vi "Write_LS_Data_without_LS370.vi"(1 "In":T1={"Time"=[], "LI1CH1"=[], "LI1CH2"=[], "LI2CH1"=[], "LI2CH2"=[], "LI3CH1"=[], "LI3CH2"=[], "Field"=[], "N_Level"=[], "H_Level"=[], "Heat_370"=[], "Sorb_Heat"=[], "Still_Heat"=[], "Capacity"=[], "Loss"=[], "Magnet_Temperature"=[], "Lam_Pressure"=[], "Lam_NValve"=[], "370-T1"=[], "370-T2"=[], "370-T3"=[], "370-T4"=[], "370-T5"=[], "370-R1"=[], "370-R2"=[], "370-R3"=[], "370-R4"=[], "370-R5"=[], "372-T1"=[], "372-T2"=[], "372-T3"=[], "372-T4"=[], "372-T5"=[], "372-T6"=[], "372-R1"=[], "372-R2"=[], "372-R3"=[], "372-R4"=[], "372-R5"=[], "372-R6"=[], "Nada"=[nan], "K2440_Res"=[], "K2440_Current"=[], "VTI_Heater"=[], "VTI_NValve"=[], "LS340_Heater"=[], "K6221_Amplitude"=[], "K6221_Frequency"=[], "Cond_Pressure"=[], "Still_Pressure"=[], "FP_Out_Pressure"=[], "Dump_Pressure"=[], "V1"=[], "V2"=[], "V4"=[], "V5"=[], "V9"=[], "Forepump"=[], "Compressor"=[], "K6221_Offset"=[], "BoxTemp"=[], "By"=[], "Bz"=[], "Phi"=[], "heater-recond (%)"=[], "Dewar Pressure "=[], "JT-SP-Control"=[], "350 T1"=[], "350 T2"=[], "350 T3"=[], "350 T4"=[], "350 R1"=[], "350 R2"=[], "350 R3"=[], "350 R4"=[], "Angle"=[], "VTI CH1"=[], "VTI CH2"=[], "VTI CH3"=[], "ColdTrap"=[], "Mischer Pot"=[], "G1 (mbar)"=[], "G3 (mbar) "=[], "G4 (mbar)"=[], "IVC (mbar)"=[], "P2 (mbar) "=[], "Pot mischer (mbar)"=[], "AVS Control Channel (K)"=[], "AVS Control Channel (RES)"=[], "AVS  Channel 5 (RES) "=[], "LI3CH3"=[], "LI3CH4"=[], "LI1CH3"=[], "LI1CH4"=[], "LI2CH3"=[], "LI2CH4"=[], "Volt"=[], "Watt"=[], "Torque Angle"=[], "Dewar heater (W)"=[], "PSU Voltage"=[], "Turbopump"=[], "372-R7"=[], "372-T7"=[], "SIM921 Ch1"=[]}) -> (0 "Out":T1={"Time"=[], "LI1CH1"=[], "LI1CH2"=[], "LI2CH1"=[], "LI2CH2"=[], "LI3CH1"=[], "LI3CH2"=[], "Field"=[], "N_Level"=[], "H_Level"=[], "Heat_370"=[], "Sorb_Heat"=[], "Still_Heat"=[], "Capacity"=[], "Loss"=[], "Magnet_Temperature"=[], "Lam_Pressure"=[], "Lam_NValve"=[], "370-T1"=[], "370-T2"=[], "370-T3"=[], "370-T4"=[], "370-T5"=[], "370-R1"=[], "370-R2"=[], "370-R3"=[], "370-R4"=[], "370-R5"=[], "372-T1"=[], "372-T2"=[], "372-T3"=[], "372-T4"=[], "372-T5"=[], "372-T6"=[], "372-R1"=[], "372-R2"=[], "372-R3"=[], "372-R4"=[], "372-R5"=[], "372-R6"=[], "Nada"=[nan], "K2440_Res"=[], "K2440_Current"=[], "VTI_Heater"=[], "VTI_NValve"=[], "LS340_Heater"=[], "K6221_Amplitude"=[], "K6221_Frequency"=[], "Cond_Pressure"=[], "Still_Pressure"=[], "FP_Out_Pressure"=[], "Dump_Pressure"=[], "V1"=[], "V2"=[], "V4"=[], "V5"=[], "V9"=[], "Forepump"=[], "Compressor"=[], "K6221_Offset"=[], "BoxTemp"=[], "By"=[], "Bz"=[], "Phi"=[], "heater-recond (%)"=[], "Dewar Pressure "=[], "JT-SP-Control"=[], "350 T1"=[], "350 T2"=[], "350 T3"=[], "350 T4"=[], "350 R1"=[], "350 R2"=[], "350 R3"=[], "350 R4"=[], "Angle"=[], "VTI CH1"=[], "VTI CH2"=[], "VTI CH3"=[], "ColdTrap"=[], "Mischer Pot"=[], "G1 (mbar)"=[], "G3 (mbar) "=[], "G4 (mbar)"=[], "IVC (mbar)"=[], "P2 (mbar) "=[], "Pot mischer (mbar)"=[], "AVS Control Channel (K)"=[], "AVS Control Channel (RES)"=[], "AVS  Channel 5 (RES) "=[], "LI3CH3"=[], "LI3CH4"=[], "LI1CH3"=[], "LI1CH4"=[], "LI2CH3"=[], "LI2CH4"=[], "Volt"=[], "Watt"=[], "Torque Angle"=[], "Dewar heater (W)"=[], "PSU Voltage"=[], "Turbopump"=[], "372-R7"=[], "372-T7"=[], "SIM921 Ch1"=[]})   [LabVIEW 2019]
uses:
  Global/Global Variables/System Monitor Cluster.ctl
  Global/Global Variables/Data_Display_global.vi
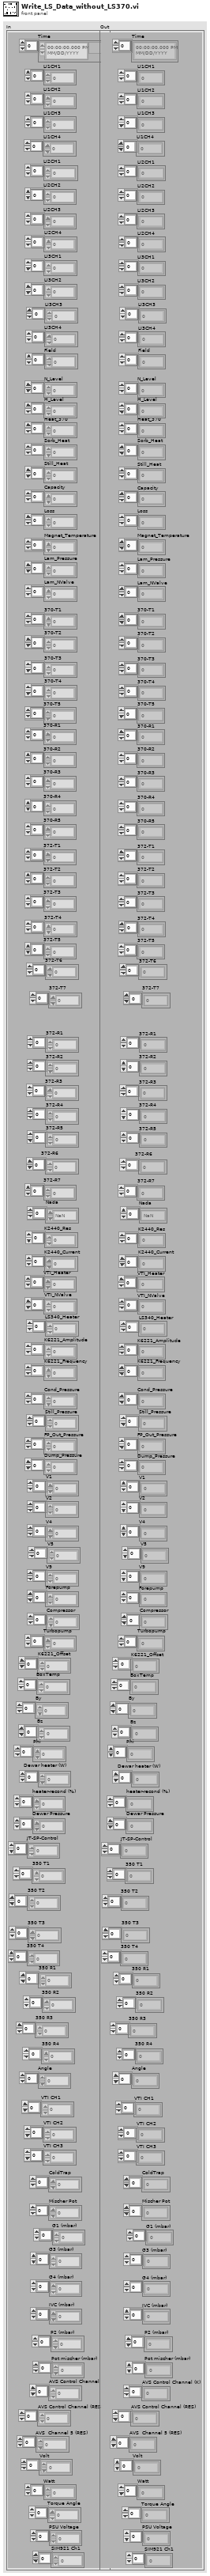
[diagram p1: front panel]
types:
  T1 = typedef "System Monitor Cluster.ctl" = cluster{"Time":timestamp[], "LI1CH1":dbl[], "LI1CH2":dbl[], "LI2CH1":dbl[], "LI2CH2":dbl[], "LI3CH1":dbl[], "LI3CH2":dbl[], "Field":dbl[], "N_Level":dbl[], "H_Level":dbl[], "Heat_370":dbl[], "Sorb_Heat":dbl[], "Still_Heat":dbl[], "Capacity":dbl[], "Loss":dbl[], "Magnet_Temperature":dbl[], "Lam_Pressure":dbl[], "Lam_NValve":dbl[], "370-T1":dbl[], "370-T2":dbl[], "370-T3":dbl[], "370-T4":dbl[], "370-T5":dbl[], "370-R1":dbl[], "370-R2":dbl[], "370-R3":dbl[], "370-R4":dbl[], "370-R5":dbl[], "372-T1":dbl[], "372-T2":dbl[], "372-T3":dbl[], "372-T4":dbl[], "372-T5":dbl[], "372-T6":dbl[], "372-R1":dbl[], "372-R2":dbl[], "372-R3":dbl[], "372-R4":dbl[], "372-R5":dbl[], "372-R6":dbl[], "Nada":dbl[], "K2440_Res":dbl[], "K2440_Current":dbl[], "VTI_Heater":dbl[], "VTI_NValve":dbl[], "LS340_Heater":dbl[], "K6221_Amplitude":dbl[], "K6221_Frequency":dbl[], "Cond_Pressure":dbl[], "Still_Pressure":dbl[], "FP_Out_Pressure":dbl[], "Dump_Pressure":dbl[], "V1":dbl[], "V2":dbl[], "V4":dbl[], "V5":dbl[], "V9":dbl[], "Forepump":dbl[], "Compressor":dbl[], "K6221_Offset":dbl[], "BoxTemp":dbl[], "By":dbl[], "Bz":dbl[], "Phi":dbl[], "heater-recond (%)":dbl[], "Dewar Pressure ":dbl[], "JT-SP-Control":dbl[], "350 T1":dbl[], "350 T2":dbl[], "350 T3":dbl[], "350 T4":dbl[], "350 R1":dbl[], "350 R2":dbl[], "350 R3":dbl[], "350 R4":dbl[], "Angle":dbl[], "VTI CH1":dbl[], "VTI CH2":dbl[], "VTI CH3":dbl[], "ColdTrap":dbl[], "Mischer Pot":dbl[], "G1 (mbar)":dbl[], "G3 (mbar) ":dbl[], "G4 (mbar)":dbl[], "IVC (mbar)":dbl[], "P2 (mbar) ":dbl[], "Pot mischer (mbar)":dbl[], "AVS Control Channel (K)":dbl[], "AVS Control Channel (RES)":dbl[], "AVS  Channel 5 (RES) ":dbl[], "LI3CH3":dbl[], "LI3CH4":dbl[], "LI1CH3":dbl[], "LI1CH4":dbl[], "LI2CH3":dbl[], "LI2CH4":dbl[], "Volt":dbl[], "Watt":dbl[], "Torque Angle":dbl[], "Dewar heater (W)":dbl[], "PSU Voltage":dbl[], "Turbopump":dbl[], "372-R7":dbl[], "372-T7":dbl[], "SIM921 Ch1":dbl[]}
  T2 = typedef "LS372_read_only-Cluster.ctl" = cluster{"LS372-T1":dbl, "LS372 -T2":dbl, "LS372-T4":dbl, "LS372-T5":dbl, "LS372-T6":dbl, "LS372-R1 ":dbl, "LS372-R2":dbl, "LS372-R3 ":dbl, "LS372-R4 \n\n\n\n":dbl, "LS372-R5":dbl, "LS372-R6 ":dbl, "LS372-T3":dbl, "Update Lakeshores":bool}
  T3 = typedef "LS350-cluster.ctl" = cluster{"Setpoint":dbl, "Heater Output":dbl, "Setpoint control":dbl, "Enable Setpoint":bool, "LS350 T1":dbl, "LS350 T2":dbl, "LS350 T3":dbl, "LS350 T4":dbl, "LS350 R1":dbl, "LS350 R2":dbl, "LS350 R3":dbl, "LS350 R4":dbl}
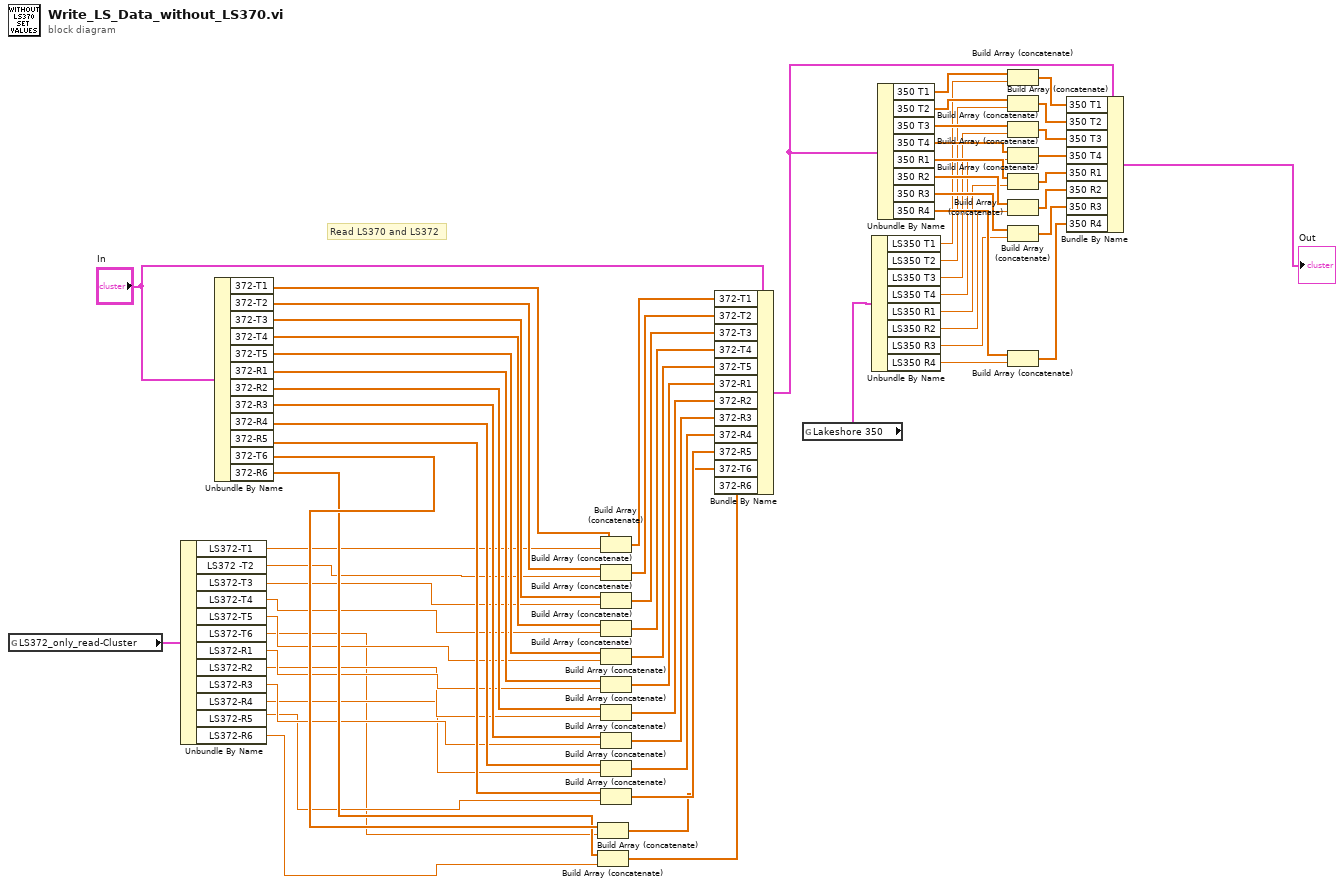
[diagram p0: block diagram]
diagram:
  # "Read LS370 and LS372"
  n1 = global read "Data_Display_global.vi" "LS372_only_read-Cluster"() -> (w13:T2)
  n2 = Unbundle By Name(w13) -> ("LS372-T1"=w12:dbl, "LS372 -T2"=w11:dbl, "LS372-T3"=w10:dbl, "LS372-T4"=w9:dbl, "LS372-T5"=w8:dbl, "LS372-T6"=w1:dbl, "LS372-R1"=w7:dbl, "LS372-R2"=w6:dbl, "LS372-R3"=w5:dbl, "LS372-R4"=w4:dbl, "LS372-R5"=w3:dbl, "LS372-R6"=w2:dbl)
  n3 = Unbundle By Name("In") -> ("372-T1"=w65:dbl[], "372-T2"=w64:dbl[], "372-T3"=w63:dbl[], "372-T4"=w62:dbl[], "372-T5"=w61:dbl[], "372-R1"=w60:dbl[], "372-R2"=w59:dbl[], "372-R3"=w58:dbl[], "372-R4"=w57:dbl[], "372-R5"=w56:dbl[], "372-T6"=w44:dbl[], "372-R6"=w43:dbl[])
  n4 = Build Array (concatenate)(w44, w1) -> (w42:dbl[])
  n5 = Build Array (concatenate)(w43, w2) -> (w41:dbl[])
  n6 = Build Array (concatenate)(w65, w12) -> (w55:dbl[])
  n7 = Build Array (concatenate)(w64, w11) -> (w54:dbl[])
  n8 = Build Array (concatenate)(w63, w10) -> (w53:dbl[])
  n9 = Build Array (concatenate)(w62, w9) -> (w52:dbl[])
  n10 = Build Array (concatenate)(w61, w8) -> (w51:dbl[])
  n11 = Build Array (concatenate)(w60, w7) -> (w50:dbl[])
  n12 = Build Array (concatenate)(w59, w6) -> (w49:dbl[])
  n13 = Build Array (concatenate)(w58, w5) -> (w45:dbl[])
  n14 = Build Array (concatenate)(w57, w4) -> (w48:dbl[])
  n15 = Build Array (concatenate)(w56, w3) -> (w47:dbl[])
  n16 = Bundle By Name(cluster="In", "372-T1"=w55, "372-T2"=w54, "372-T3"=w53, "372-T4"=w52, "372-T5"=w51, "372-R1"=w50, "372-R2"=w49, "372-R3"=w45, "372-R4"=w48, "372-R5"=w47, "372-T6"=w42, "372-R6"=w41) -> (w23:T1)
  n17 = global read "Data_Display_global.vi" "Lakeshore 350"() -> (w40:T3)
  n18 = Unbundle By Name(w40) -> ("LS350 T1"=w24:dbl, "LS350 T2"=w25:dbl, "LS350 T3"=w26:dbl, "LS350 T4"=w27:dbl, "LS350 R1"=w28:dbl, "LS350 R2"=w29:dbl, "LS350 R3"=w30:dbl, "LS350 R4"=w31:dbl)
  n19 = Unbundle By Name(w23) -> ("350 T1"=w39:dbl[], "350 T2"=w38:dbl[], "350 T3"=w37:dbl[], "350 T4"=w36:dbl[], "350 R1"=w35:dbl[], "350 R2"=w34:dbl[], "350 R3"=w33:dbl[], "350 R4"=w32:dbl[])
  n20 = Build Array (concatenate)(w39, w24) -> (w21:dbl[])
  n21 = Build Array (concatenate)(w38, w25) -> (w20:dbl[])
  n22 = Build Array (concatenate)(w37, w26) -> (w19:dbl[])
  n23 = Build Array (concatenate)(w36, w27) -> (w18:dbl[])
  n24 = Build Array (concatenate)(w35, w28) -> (w17:dbl[])
  n25 = Build Array (concatenate)(w34, w29) -> (w16:dbl[])
  n26 = Build Array (concatenate)(w33, w30) -> (w15:dbl[])
  n27 = Build Array (concatenate)(w32, w31) -> (w14:dbl[])
  n28 = Bundle By Name(cluster=w23, "350 T1"=w21, "350 T2"=w20, "350 T3"=w19, "350 T4"=w18, "350 R1"=w17, "350 R2"=w16, "350 R3"=w15, "350 R4"=w14) -> (→"Out":T1)
